vi "FVI_Trajectiore_Swerve4vitesse.vi"(0 "Vx":dbl, 5 "Vy":dbl, 7 "Omega":dbl, 12 "Distance":dbl) -> (4 "SwerveDrive":T1)   [LabVIEW 2018]
uses:
  SwerveDrive.ctl
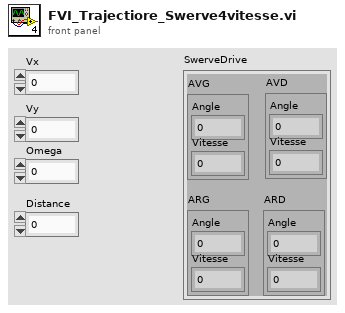
[diagram p1: front panel]
types:
  T1 = typedef "SwerveDrive.ctl" = cluster{"AVD":cluster{"Angle":dbl, "Vitesse":dbl}, "AVG":cluster{"Angle":dbl, "Vitesse":dbl}, "ARG":cluster{"Angle":dbl, "Vitesse":dbl}, "ARD":cluster{"Angle":dbl, "Vitesse":dbl}}
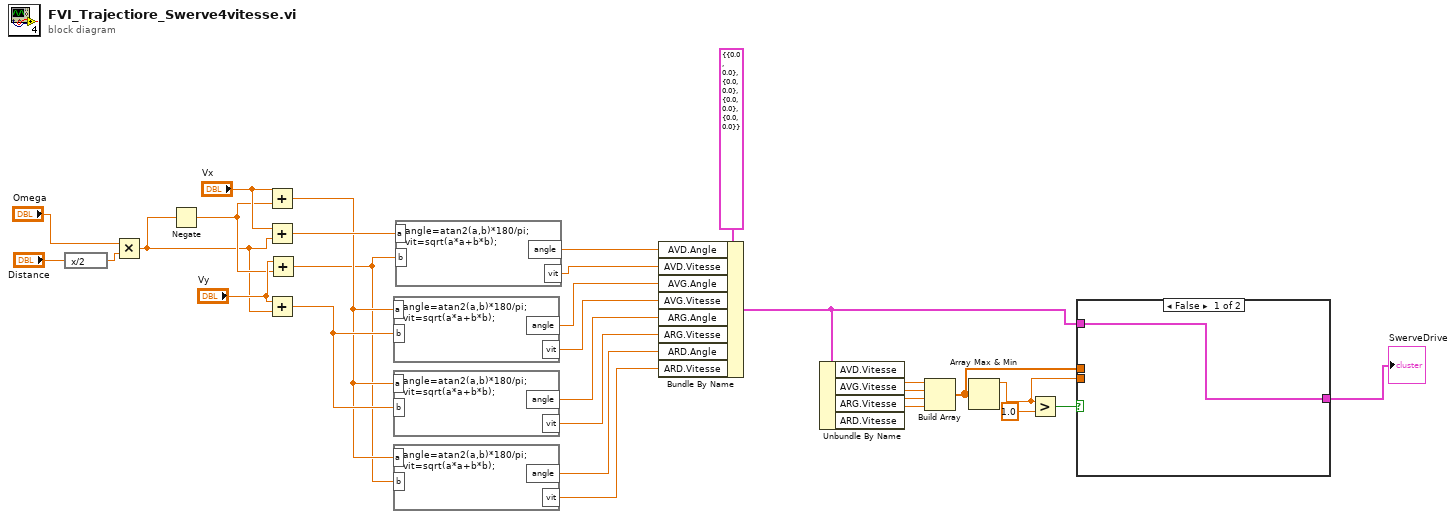
[diagram p0: block diagram]
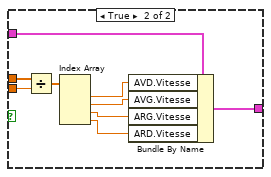
[diagram p2: hidden frame]
diagram:
  n1 = expression code="x/2"("Distance") -> (w28:dbl)
  n2 = Multiply(x="Omega", y=w28) -> (x*y=w23:dbl)
  n3 = Negate(x=w23) -> (-x=w24:dbl)
  n4 = Add(x="Vx", y=w24) -> (x+y=w18:dbl)
  n5 = Add(x="Vx", y=w23) -> (x+y=w22:dbl)
  n6 = Add(x="Vy", y=w23) -> (x+y=w19:dbl)
  n7 = Add(x="Vy", y=w24) -> (x+y=w17:dbl)
  n8 = formula code="angle=atan2(a,b)*180/pi;\nvit=sqrt(a*a+b*b);"("a"=w18, "b"=w19) -> ("angle"=w16:dbl, "vit"=w15:dbl)
  n9 = formula code="angle=atan2(a,b)*180/pi;\nvit=sqrt(a*a+b*b);"("a"=w18, "b"=w19) -> ("angle"=w14:dbl, "vit"=w13:dbl)
  n10 = formula code="angle=atan2(a,b)*180/pi;\nvit=sqrt(a*a+b*b);"("a"=w18, "b"=w17) -> ("angle"=w12:dbl, "vit"=w11:dbl)
  n11 = formula code="angle=atan2(a,b)*180/pi;\nvit=sqrt(a*a+b*b);"("a"=w22, "b"=w17) -> ("angle"=w21:dbl, "vit"=w20:dbl)
  n12 = Bundle By Name(cluster=T1 {"AVD"={"Angle"=0.0, "Vitesse"=0.0}, "AVG"={"Angle"=0.0, "Vitesse"=0.0}, "ARG"={"Angle"=0.0, "Vitesse"=0.0}, "ARD"={"Angle"=0.0, "Vitesse"=0.0}} ("SwerveDrive"), "AVD.Angle"=w21, "AVD.Vitesse"=w20, "AVG.Angle"=w16, "AVG.Vitesse"=w15, "ARG.Angle"=w14, "ARG.Vitesse"=w13, "ARD.Angle"=w12, "ARD.Vitesse"=w11) -> (w2:T1)
  n13 = Unbundle By Name(w2) -> ("AVD.Vitesse"=w10:dbl, "AVG.Vitesse"=w7:dbl, "ARG.Vitesse"=w8:dbl, "ARD.Vitesse"=w9:dbl)
  n14 = Build Array(w10, w7, w8, w9) -> (w4:dbl[])
  n15 = Array Max & Min(array=w4) -> (max value=w3:dbl)  [unwired: 3 out]
  n16 = Greater?(x=w3, y=1.0) -> (0:w5:bool)
  n17 = case shown="False" w5 {
    tunnel: w4 -> [_ w40]
    tunnel: w3 -> [_ w39]
    tunnel: w2 -> [w31 w33]
    tunnel: [w31 w32] -> w1
    frame False {
    }
    frame True {
      n18 = Divide(x=w40, y=w39) -> (x/y=w38:dbl[])
      n19 = Index Array(array=w38) -> (element #1=w37:dbl, element #2=w36:dbl, element #3=w35:dbl, element #4=w34:dbl)  [unwired: 4 in]
      n20 = Bundle By Name(cluster=w33, "AVD.Vitesse"=w37, "AVG.Vitesse"=w36, "ARG.Vitesse"=w35, "ARD.Vitesse"=w34) -> (w32:T1)
    }
  }
  "SwerveDrive" <- w1
